vi "DrawSegment__slk_mt.vi"(4 "color":u32(colorbox)=32639, 6 "pen":T1={"Width"=1, "Style"=enum."Dot"}, 8 "error in (no error)":errorcluster, 10 "joints":cluster{"X":i32, "Y":i32}[](array[cluster]), 11 "view in":refnum<class "View__slk_mt.lvclass">) -> (0 "error out":errorcluster, 3 "view out":refnum<class "View__slk_mt.lvclass">)   [LabVIEW 2013, in "Lazyboots Menu Tool.lvlib" / "View__slk_mt.lvclass"]
doc: "Draws segment to view object."
uses:
  View__slk_mt.lvclass
panel:
  # "DrawSegment__slk_mt.vi\nDraws segment to view object.\n\nNOTICE -- YOU MUST LEAVE THIS NOTICE IN PLACE.\n\nCopyright (c) 2011, LIANG LIU Shawn.Liu.cn@gmail.com\nAll rights reserved.\n\nRedistribution and use in source and binary forms, with or without modification, are permitted provided that the following conditions are met:\n-Redistributions of source code must retain the above copyright notice, this list of conditions and the following disclaimer.\n-Redistributions in binary form must reproduce the above copyright notice, this list of conditions and the following disclaimer in the documentation and/or other materials provided with the distribution.\n-Neither the name of the eLp nor the names of its contributors may be used to endorse or promote products derived from this software without specific prior written permission.\n\nTHIS SOFTWARE IS PROVIDED BY THE COPYRIGHT HOLDERS AND CONTRIBUTORS \"AS IS\" AND ANY EXPRESS OR IMPLIED WARRANTIES, INCLUDING, BUT NOT LIMITED TO, THE IMPLIED WARRANTIES OF MERCHANTABILITY AND FITNESS FOR A PARTICULAR PURPOSE ARE DISCLAIMED. IN NO EVENT SHALL THE COPYRIGHT HOLDER OR CONTRIBUTORS BE LIABLE FOR ANY DIRECT, INDIRECT, INCIDENTAL, SPECIAL, EXEMPLARY, OR CONSEQUENTIAL DAMAGES (INCLUDING, BUT NOT LIMITED TO, PROCUREMENT OF SUBSTITUTE GOODS OR SERVICES; LOSS OF USE, DATA, OR PROFITS; OR BUSINESS INTERRUPTION) HOWEVER CAUSED AND ON ANY THEORY OF LIABILITY, WHETHER IN CONTRACT, STRICT LIABILITY, OR TORT (INCLUDING NEGLIGENCE OR OTHERWISE) ARISING IN ANY WAY OUT OF THE USE OF THIS SOFTWARE, EVEN IF ADVISED OF THE POSSIBILITY OF SUCH DAMAGE."
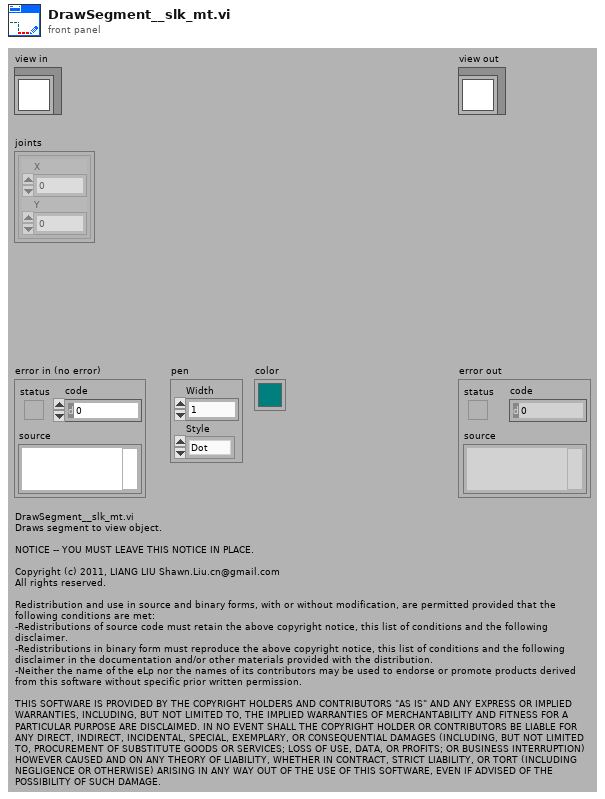
[diagram p1: front panel]
types:
  T1 = cluster{"Width":u16, "Style":enum32{"Solid", "Dash", "Dot", "DashDot", "DashDotDot"}}
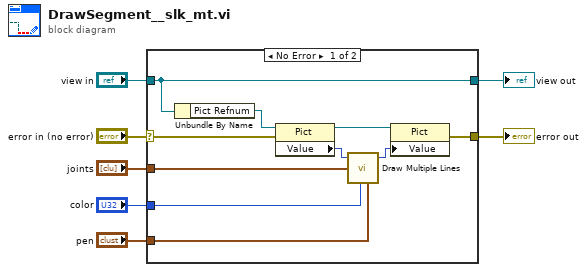
[diagram p0: block diagram]
diagram:
  n1 = case shown="No Error" "error in (no error)" {
    selector: "error in (no error)" -> [w11 w19]
    tunnel: [w12 w19] -> w6
    tunnel: [w17 w18] -> w4
    tunnel: "view in" -> [w17 w18]
    tunnel: "joints" -> [w10 _]
    tunnel: "color" -> [w9 _]
    tunnel: "pen" -> [w8 _]
    frame No Error {
      n2 = Unbundle By Name(w17) -> ("Pict Refnum"=w16:refnum<vi>)
      n3 = property class="Pict"(reference=w16, error in=w11) -> (reference out=w15:refnum<vi>, "Value"=w14:picture)  [unwired: 1 out]
      n4 = call <vilib>:"Draw Multiple Lines.vi"("picture"=w14, "line endpoints"=w10, "color(black)"=w9, "pen"=w8) -> ("new picture"=w13:picture)  [unwired: 5 in]
      n5 = property class="Pict"(reference=w15, "Value"=w13) -> (error out=w12:errorcluster)  [unwired: 1 in, 1 out]
    }
    frame Error {
    }
  }
  "error out" <- w6
  "view out" <- w4
